vi "Obtain-DBAL-Queue.vi"() -> (6 "DBAL-Queue":refnum<queue>)   [LabVIEW 2020]
doc: "Obtain a queue for DBAL service"
uses:
  controls/DBAL_Command.ctl
  controls/DBAL-commands.ctl
  DBAL.lvclass
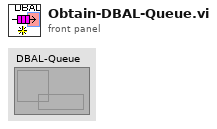
[diagram p1: front panel]
types:
  T1 = typedef "Sgraph_lib_V1.lvlib/DBAL.lvclass/DBAL_Command.ctl" = cluster{"Source":string, "Command":T2, "Time Stamp":timestamp, "data":variant}
  T2 = typedef "Sgraph_lib_V1.lvlib/DBAL.lvclass/DBAL-commands.ctl" = enum16{"idle", "SavePAQdata", "ExitService"}
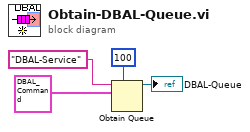
[diagram p0: block diagram]
diagram:
  n1 = Obtain Queue(max queue size (-1, unlimited)=100, name (unnamed)="DBAL-Service", element data type=T1 {"Source"="", "Command"=enum."idle", "Time Stamp"=timestamp(0 s since 1904-01-01), "data"=variant} ("Cluster")) -> (queue out=→"DBAL-Queue":refnum<queue>)  [unwired: 2 in, 2 out]
